vi "Close Connection with CD.vi"(8 "error in":errorcluster, 11 "Comm Ref":T1) -> (0 "error out":errorcluster)   [LabVIEW 2013, in "PID Control Host API.lvlib"]
uses:
  PID Control Host API.lvlib
  <vilib>/NI Veristand/Execution/CustomDevice/Custom Device Ref.ctl
  NationalInstruments.VeriStand.ClientAPI
  <vilib>/NI VeriStand/Execution/CustomDevice/NI_VS Custom Device ExecutionAPI.lvlib
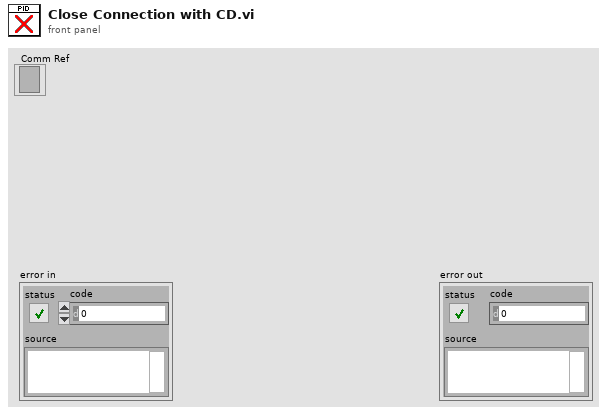
[diagram p1: front panel]
types:
  T1 = typedef "NI_VS Custom Device ExecutionAPI.lvlib/Custom Device Ref.ctl" = refnum<k24>
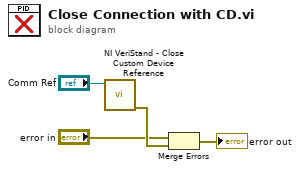
[diagram p0: block diagram]
diagram:
  n1 = call <vilib>:"NI VeriStand - Close Custom Device Reference.vi"("Custom Device"="Comm Ref") -> ("error out"=w4:errorcluster)  [unwired: 10 in]
  n2 = Merge Errors("error in", w4) -> (→"error out":errorcluster)
